vi "load.vi"(8 "error in (no error)":errorcluster, 10 "Node":refnum<k20>, 11 "HP83712B_RF_Generator in":refnum<class "HP83712B_RF_Generator.lvclass">) -> (0 "error out":errorcluster, 2 "node out":refnum<k20>, 3 "HP83712B_RF_Generator out":refnum<class "HP83712B_RF_Generator.lvclass">)   [LabVIEW 2013, in "HP83712B_RF_Generator.lvclass"]
uses:
  HP83712B_RF_Generator.lvclass
  RF_Generator_settings.ctl
  HP83712B_RF_Generator.lvclass/HP83712B_RF_Generator.ctl
  <vilib>/xml/Close Reference(Node).vi
  <vilib>/xml/NI_XML.lvlib
  <resource>/objmgr/DOMUserDefRef.rc
  GPIB.lvclass
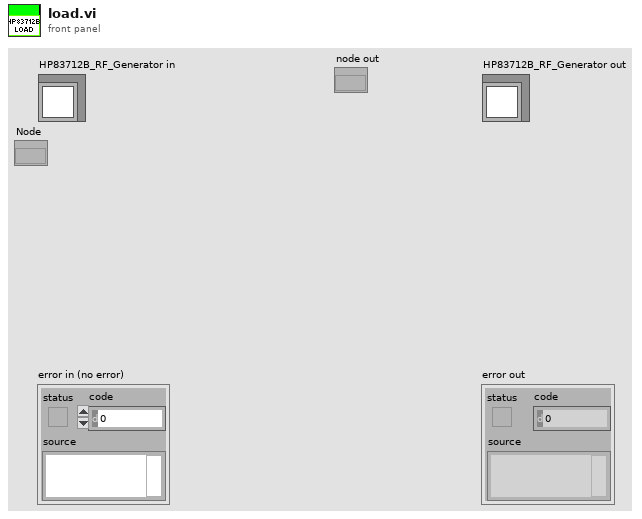
[diagram p1: front panel]
types:
  T1 = typedef "GPIB.lvclass/RF_Generator_settings.ctl" = cluster{"Enable":bool, "Description":string, "GPIB channel #":u8, "Frequency (MHz)":dbl, "Power (dBm)":dbl}
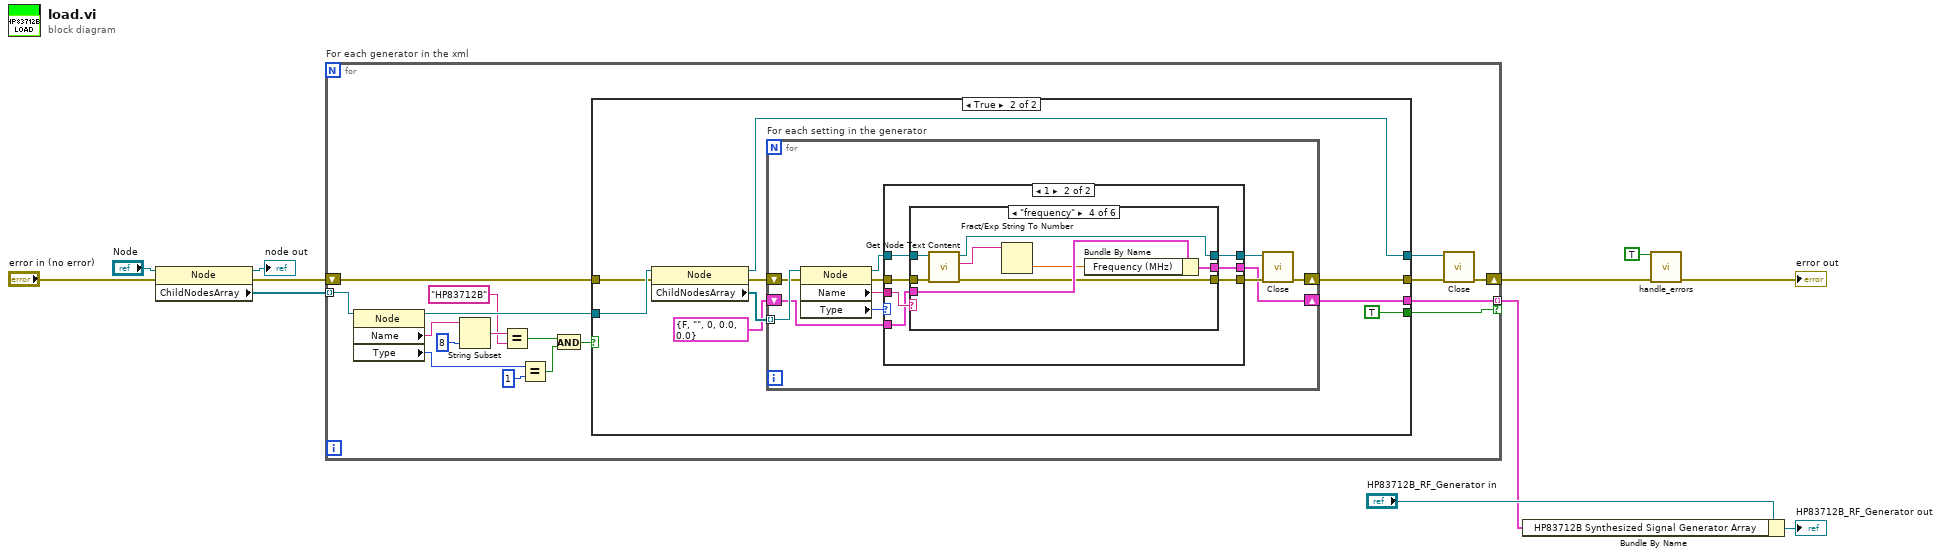
[diagram p0: block diagram]
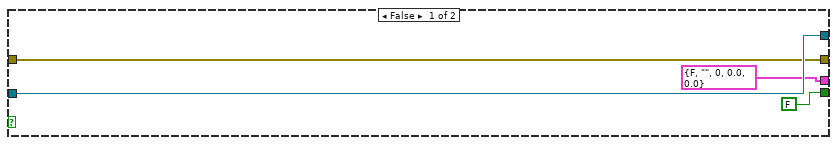
[diagram p2: hidden frame]
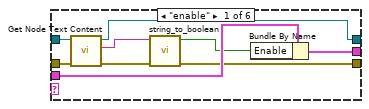
[diagram p4: hidden frame]
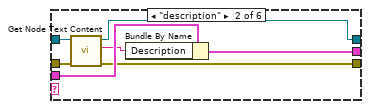
[diagram p5: hidden frame]
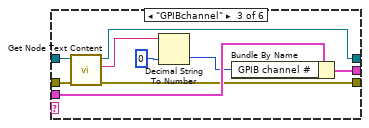
[diagram p6: hidden frame]
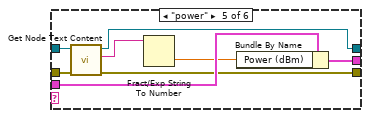
[diagram p7: hidden frame]
diagram:
  n1 = property class="Node"(reference="Node", error in="error in (no error)") -> (reference out=→"node out":refnum<k20>, error out=w4:errorcluster, "ChildNodesArray"=w5:refnum<k20>[])
  n2 = for "For each generator in the xml" {
    tunnel: w5 -> [w22] mode=indexing
    shift-right: [w25] -> w3
    shift-left: w4 -> [w28]
    tunnel: [w24] -> w9 mode=indexing if=w23
    n3 = property class="Node"(reference=w22) -> (reference out=w21:refnum<k20>, "Name"=w17:string, "Type"=w20:i32)  [unwired: 1 in, 1 out]
    n4 = String Subset(string=w17, length (rest)=8 ("length (rest)")) -> (substring=w15:string)  [unwired: 1 in]
    n5 = Equal?(x=w15, y="HP83712B") -> (x = y?=w13:bool)
    n6 = Equal?(x=w20, y=1) -> (x = y?=w18:bool)
    n7 = And(x=w13, y=w18) -> (x .and. y?=w12:bool)
    n8 = case shown="True" w12 {
      tunnel: w21 -> [w32 w41]
      tunnel: w28 -> [w31 w40]
      tunnel: [w32 w37] -> w27
      tunnel: [w31 w36] -> w26
      tunnel: [T1 {"Enable"=FALSE, "Description"="", "GPIB channel #"=0, "Frequency (MHz)"=0.0, "Power (dBm)"=0.0} ("Cluster") w35] -> w24
      tunnel: [FALSE TRUE] -> w23
      frame False {
      }
      frame True {
        n9 = property class="Node"(reference=w41, error in=w40) -> (reference out=w37:refnum<k20>, error out=w38:errorcluster, "ChildNodesArray"=w39:refnum<k20>[])
        n10 = for "For each setting in the generator" {
          shift-right: [w45] -> w36
          shift-left: w38 -> [w49]
          tunnel: w39 -> [w52] mode=indexing
          shift-right: [w43] -> w35
          shift-left: T1 {"Enable"=FALSE, "Description"="", "GPIB channel #"=0, "Frequency (MHz)"=0.0, "Power (dBm)"=0.0} ("Cluster") -> [w44]
          n11 = property class="Node"(reference=w52, error in=w49) -> (reference out=w47:refnum<k20>, error out=w50:errorcluster, "Name"=w51:string, "Type"=w42:i32)
          n12 = case shown="1" w42 {
            tunnel: w51 -> [_ w62]
            tunnel: w50 -> [w54 w61]
            tunnel: [w55 w60] -> w48
            tunnel: w47 -> [w55 w59]
            tunnel: [w54 w58] -> w46
            tunnel: w44 -> [w53 w57]
            tunnel: [w53 w56] -> w43
            frame Default {
            }
            frame 1 {
              n13 = case shown="\"frequency\"" w62 {
                tunnel: w61 -> [w70 w77 w86 w94 w102 w106]
                tunnel: [w63 w72 w82 w90 w98 w106] -> w58
                tunnel: [w67 w73 w83 w91 w99 w105] -> w60
                tunnel: w59 -> [w71 w78 w87 w95 w103 w105]
                tunnel: w57 -> [w69 w76 w85 w93 w101 w104]
                tunnel: [w68 w75 w84 w92 w100 w104] -> w56
                frame "enable" {
                  n14 = call <vilib>:"Get Node Text Content.vi"("error in (no error)"=w70, "node in"=w71) -> ("error out"=w64:errorcluster, "node text"=w66:string, "node out"=w67:refnum<k20>)  [unwired: 7 in]
                  n15 = call "string_to_boolean.vi"("error in"=w64, "string"=w66) -> ("error out"=w63:errorcluster, "boolean"=w65:bool)  [unwired: 8 in]
                  n16 = Bundle By Name(cluster=w69, "Enable"=w65) -> (w68:T1)
                }
                frame "description" {
                  n17 = call <vilib>:"Get Node Text Content.vi"("error in (no error)"=w77, "node in"=w78) -> ("error out"=w72:errorcluster, "node text"=w74:string, "node out"=w73:refnum<k20>)  [unwired: 7 in]
                  n18 = Bundle By Name(cluster=w76, "Description"=w74) -> (w75:T1)
                }
                frame "GPIBchannel" {
                  n19 = call <vilib>:"Get Node Text Content.vi"("error in (no error)"=w86, "node in"=w87) -> ("error out"=w82:errorcluster, "node text"=w81:string, "node out"=w83:refnum<k20>)  [unwired: 7 in]
                  n20 = Decimal String To Number(string=w81, default (0L)=u8 0 ("default (0 I32)")) -> (number=w80:u8)  [unwired: 1 in, 1 out]
                  n21 = Bundle By Name(cluster=w85, "GPIB channel #"=w80) -> (w84:T1)
                }
                frame "frequency" {
                  n22 = call <vilib>:"Get Node Text Content.vi"("error in (no error)"=w94, "node in"=w95) -> ("error out"=w90:errorcluster, "node text"=w89:string, "node out"=w91:refnum<k20>)  [unwired: 7 in]
                  n23 = Fract/Exp String To Number(string=w89) -> (number=w88:dbl)  [unwired: 3 in, 1 out]
                  n24 = Bundle By Name(cluster=w93, "Frequency (MHz)"=w88) -> (w92:T1)
                }
                frame "power" {
                  n25 = call <vilib>:"Get Node Text Content.vi"("error in (no error)"=w102, "node in"=w103) -> ("error out"=w98:errorcluster, "node text"=w97:string, "node out"=w99:refnum<k20>)  [unwired: 7 in]
                  n26 = Fract/Exp String To Number(string=w97) -> (number=w96:dbl)  [unwired: 3 in, 1 out]
                  n27 = Bundle By Name(cluster=w101, "Power (dBm)"=w96) -> (w100:T1)
                }
                frame Default {
                }
              }
            }
          }
          n28 = call-poly <vilib>:"Close.vi"("error in (no error)"=w46, "node"=w48) -> ("error out"=w45:errorcluster)  [unwired: 7 in]
        }
      }
    }
    n29 = call-poly <vilib>:"Close.vi"("error in (no error)"=w26, "node"=w27) -> ("error out"=w25:errorcluster)  [unwired: 7 in]
  }
  n30 = Bundle By Name(cluster="HP83712B_RF_Generator in", "HP83712B Synthesized Signal Generator Array"=w9) -> (→"HP83712B_RF_Generator out":refnum<class "HP83712B_RF_Generator.lvclass">)
  n31 = call "handle_errors.vi"("Exit Operation"=TRUE, "error in (no error)"=w3) -> ("error out"=→"error out":errorcluster)  [unwired: 13 in]
